vi "AMZ_S3_APIHLP_Parse POST Multipart Object Request Parameters.vi"(7 "POST Multipart Object Request Parameters":T1, 8 "error in (no error)":errorcluster, 11 "HTTP Headers in":T5[](array[typedef])) -> (0 "error out":errorcluster, 3 "HTTP Headers":T5[](array[typedef]))   [LabVIEW 2015, in "LV Interface for Amazon S3.lvlib"]
uses:
  LV Interface for Amazon S3.lvlib
  Typedefs/AMZ_S3_HTTP Header-Value pair.ctl
  Typedefs/AMZ_S3_API_POST Multipart Object Request Parameters.ctl
  Typedefs/AMZ_S3_ACL.ctl
  Typedefs/AMZ_S3_Storage Class.ctl
  Typedefs/AMZ_S3_Object Metadata.ctl
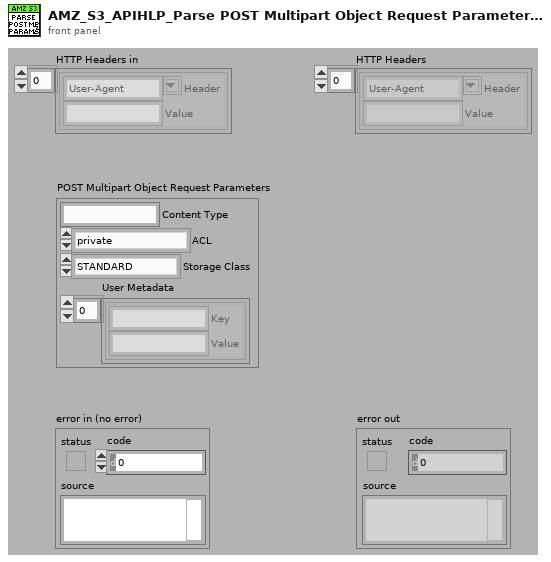
[diagram p1: front panel]
types:
  T1 = typedef "LV Interface for Amazon S3.lvlib/AMZ_S3_API_POST Multipart Object Request Parameters.ctl" = cluster{"Content Type":string, "ACL":T2, "Storage Class":T3, "User Metadata":T4[]}
  T2 = typedef "LV Interface for Amazon S3.lvlib/AMZ_S3_ACL.ctl" = enum16{"private", "public-read", "public-read-write", "aws-exec-read", "authenticated-read", "bucket-owner-read", "bucket-owner-full-control"}
  T3 = typedef "LV Interface for Amazon S3.lvlib/AMZ_S3_Storage Class.ctl" = enum16{"STANDARD", "REDUCED_REDUNDANCY"}
  T4 = typedef "LV Interface for Amazon S3.lvlib/AMZ_S3_Object Metadata.ctl" = cluster{"Key":string, "Value":string}
  T5 = typedef "LV Interface for Amazon S3.lvlib/AMZ_S3_HTTP Header-Value pair.ctl" = cluster{"Header":string, "Value":string}
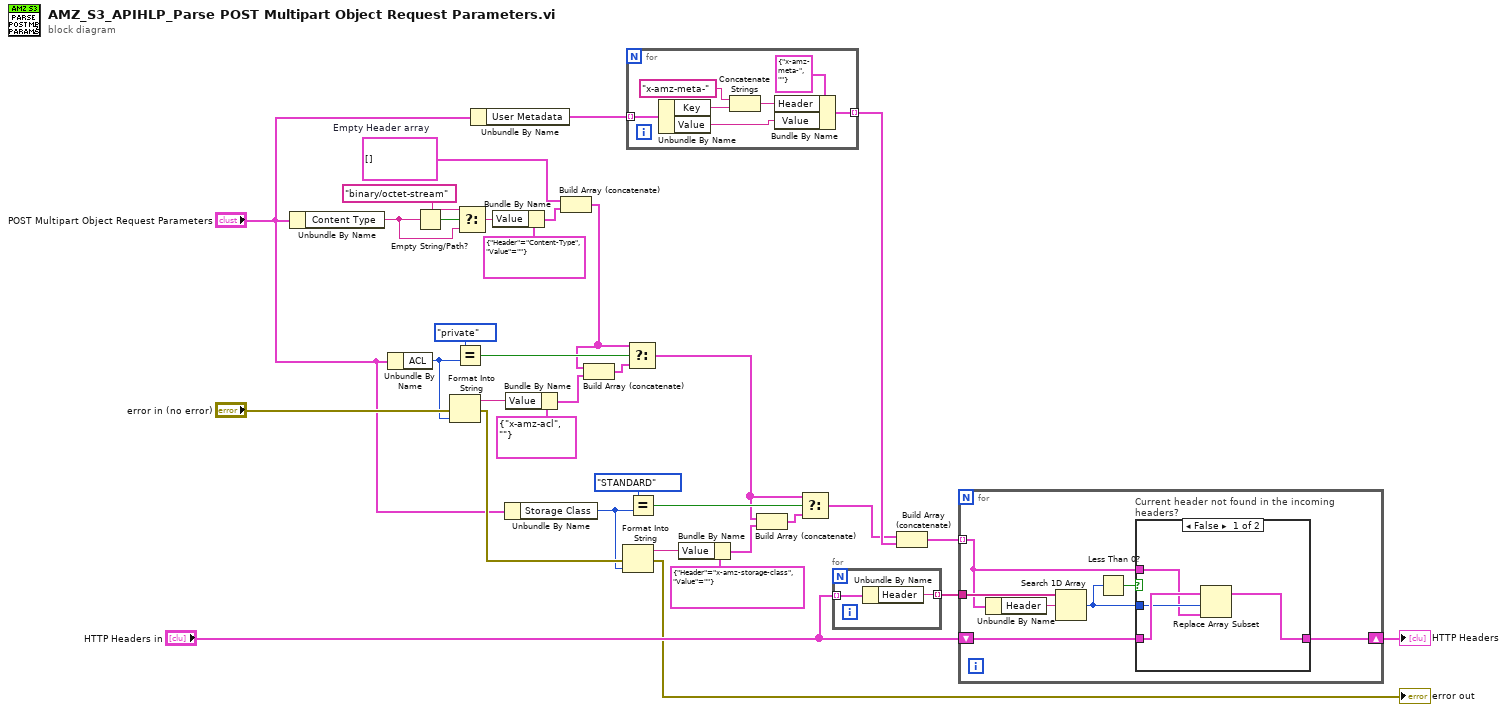
[diagram p0: block diagram]
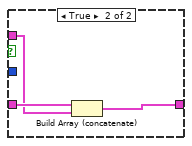
[diagram p2: hidden frame]
diagram:
  w7 = T5[] []  # Empty Header array
  n1 = Unbundle By Name("POST Multipart Object Request Parameters") -> ("Content Type"=w5:string)
  n2 = Unbundle By Name("POST Multipart Object Request Parameters") -> ("ACL"=w29:T2)
  n3 = Empty String/Path?(string/path=w5) -> (empty?=w6:bool)
  n4 = Format Into String(error in="error in (no error)", w29) -> (resulting string=w27:string, error out=w18:errorcluster)  [unwired: 2 in]
  n5 = Equal?(x=AMZ_S3_ACL."private", y=w29) -> (x = y?=w32:bool)
  n6 = Select(t="binary/octet-stream", s=w6, f=w5) -> (s? t:f=w3:string)
  n7 = Unbundle By Name("POST Multipart Object Request Parameters") -> ("User Metadata"=w15:T4[])
  n8 = Bundle By Name(cluster=T5 {"Header"="Content-Type", "Value"=""} ("HTTP Header-Value pair"), "Value"=w3) -> (w2:T5)
  n9 = Unbundle By Name("POST Multipart Object Request Parameters") -> ("Storage Class"=w17:T3)
  n10 = Bundle By Name(cluster=T5 {"Header"="x-amz-acl", "Value"=""} ("HTTP Header-Value pair"), "Value"=w27) -> (w26:T5)
  n11 = Build Array (concatenate)(w7, w2) -> (w1:T5[])
  n12 = Build Array (concatenate)(w1, w26) -> (w31:T5[])
  n13 = Format Into String(error in=w18, w17) -> (resulting string=w24:string, error out=→"error out":errorcluster)  [unwired: 2 in]
  n14 = for {
    tunnel: w15 -> [w41] mode=indexing
    tunnel: [w35] -> w14 mode=indexing
    n15 = Unbundle By Name(w41) -> ("Key"=w39:string, "Value"=w36:string)
    n16 = Concatenate Strings("x-amz-meta-", w39) -> (w37:string)
    n17 = Bundle By Name(cluster=T5 {"Header"="x-amz-meta-", "Value"=""} ("HTTP Header-Value pair"), "Header"=w37, "Value"=w36) -> (w35:T5)
  }
  n18 = Select(t=w1, s=w32, f=w31) -> (s? t:f=w19:T5[])
  n19 = Equal?(x=AMZ_S3_Storage_Class."STANDARD", y=w17) -> (x = y?=w21:bool)
  n20 = Bundle By Name(cluster=T5 {"Header"="x-amz-storage-class", "Value"=""} ("HTTP Header-Value pair"), "Value"=w24) -> (w25:T5)
  n21 = Build Array (concatenate)(w19, w25) -> (w22:T5[])
  n22 = Select(t=w19, s=w21, f=w22) -> (s? t:f=w8:T5[])
  n23 = for {
    tunnel: "HTTP Headers in" -> [w43] mode=indexing
    tunnel: [w42] -> w12 mode=indexing
    n24 = Unbundle By Name(w43) -> ("Header"=w42:string)
  }
  n25 = Build Array (concatenate)(w8, w14) -> (w13:T5[])
  n26 = for {
    tunnel: w13 -> [w46] mode=indexing
    tunnel: w12 -> [w50]
    shift-right: [w44] -> w10
    shift-left: "HTTP Headers in" -> [w45]
    n27 = Unbundle By Name(w46) -> ("Header"=w49:string)
    n28 = Search 1D Array(1D array=w50, element=w49) -> (index of element=w47:i32)  [unwired: 1 in]
    n29 = Less Than 0?(x=w47) -> (x < 0?=w48:bool)
    n30 = case "Current header not found in the incoming headers?" shown="False" w48 {
      tunnel: w47 -> [w53 _]
      tunnel: w46 -> [w52 w56]
      tunnel: w45 -> [w54 w57]
      tunnel: [w51 w55] -> w44
      frame False {
        n31 = Replace Array Subset(array=w54, new element=w52, index=w53) -> (w51:T5[])
      }
      frame True {
        n32 = Build Array (concatenate)(w57, w56) -> (w55:T5[])
      }
    }
  }
  "HTTP Headers" <- w10
